vi "GetlastDate.vi"() -> (0 "ResultLine":string, 1 "text":string, 2 "last Date":string, 3 "FRowAsArr":dbl[][](array[numeric]) format="%#_2g")   [LabVIEW 2023]
panel:
  out "result string":string
  out "Array":string[](array[string])
  out "All Officials Result":dbl[][](array[numeric])
  out "First Row":dbl[](array[numeric])
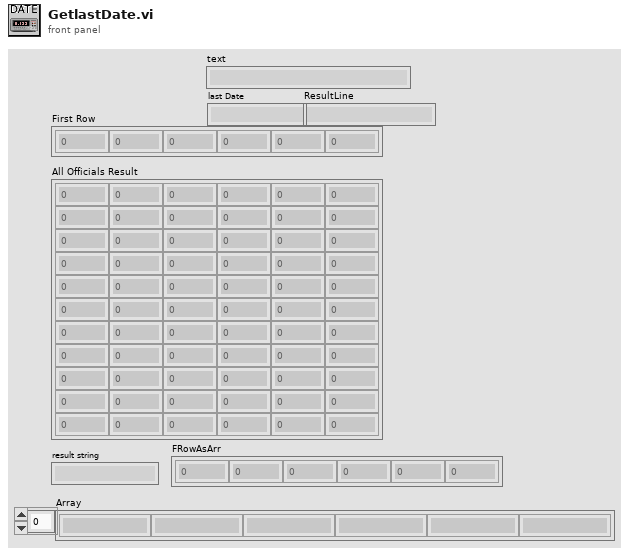
[diagram p1: front panel]
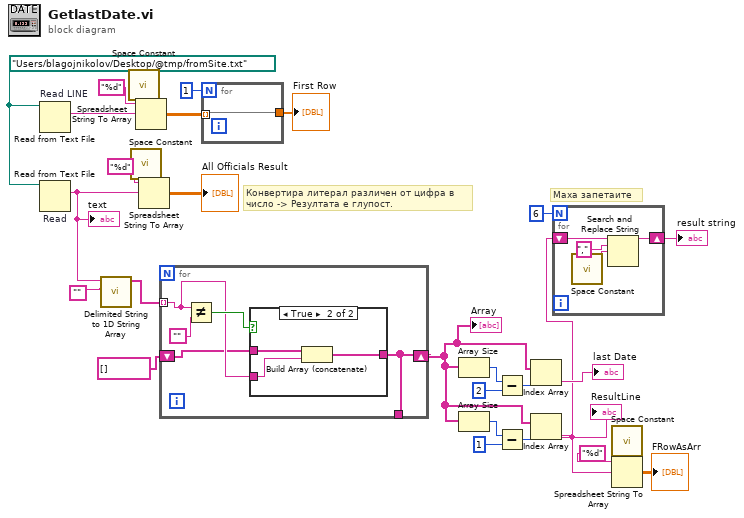
[diagram p0: block diagram]
diagram:
  w20 = path "/Users/blagojnikolov/Desktop/@tmp/fromSite.txt" ("file (use dialog)")
  # "Конвертира литерал различен от цифра в \nчисло -> Резултата е глупост."
  # "Маха запетаите"
  n1 = Read from Text File "Read LINE"(file (use dialog)=w20) -> (text=w28:string)  [unwired: 3 in, 3 out]
  n2 = Read from Text File "Read"(file (use dialog)=w20) -> (text=w18:string)  [unwired: 3 in, 3 out]
  "text" <- w18
  n3 = call <vilib>:"Delimited String to 1D String Array.vi"("delimiter"="", "delimited string"=w18) -> ("string array"=w16:string[])  [unwired: 9 in]
  n4 = call <vilib>:"Space Constant.vi"() -> ("String"=w26:string)
  n5 = call <vilib>:"Space Constant.vi"() -> ("String"=w22:string)
  n6 = Spreadsheet String To Array(delimiter (Tab)=w26, format string="%d", spreadsheet string=w28) -> (array=w25:dbl[][])  [unwired: 1 in]
  n7 = Spreadsheet String To Array(delimiter (Tab)=w22, format string="%d", spreadsheet string=w18) -> (array=→"All Officials Result":dbl[][])  [unwired: 1 in]
  n8 = for {
    tunnel: w16 -> [w31] mode=indexing
    shift-right: [w29] -> w5
    shift-left: string[] [] -> [w30]
    tunnel: [w29] -> _
    n9 = Not Equal?(x=w31, y="") -> (x != y?=w32:bool)
    n10 = case shown="True" w32 {
      tunnel: w31 -> [_ w37]
      tunnel: [w34 w36] -> w29
      tunnel: w30 -> [w34 w35]
      frame False {
      }
      frame True {
        n11 = Build Array (concatenate)(w35, w37) -> (w36:string[])
      }
    }
  }
  "Array" <- w5
  n12 = for {
    N: 1 -> [_]
    tunnel: w25 -> [w38] mode=indexing
    tunnel: [w38] -> w23
  }
  "First Row" <- w23
  n13 = Array Size(array=w5) -> (size(s)=w14:i32)
  n14 = Array Size(array=w5) -> (size(s)=w9:i32)
  n15 = Subtract(x=w14, y=2) -> (x-y=w13:i32)
  n16 = Subtract(x=w9, y=1) -> (x-y=w10:i32)
  n17 = Index Array(array=w5, index=w13) -> (element=→"last Date":string)
  n18 = Index Array(array=w5, index=w10) -> (element=w2:string)
  "ResultLine" <- w2
  n19 = for {
    N: 6 -> [_]
    shift-right: [w40] -> w1
    shift-left: w2 -> [w39]
    n20 = call <vilib>:"Space Constant.vi"() -> ("String"=w41:string)
    n21 = Search and Replace String(input string=w39, search string="," ("replace string (\"\")"), replace string=w41) -> (result string=w40:string)  [unwired: 5 in, 3 out]
  }
  "result string" <- w1
  n22 = call <vilib>:"Space Constant.vi"() -> ("String"=w8:string)
  n23 = Spreadsheet String To Array(delimiter (Tab)=w8, format string="%d", spreadsheet string=w2) -> (array=→"FRowAsArr":dbl[][])  [unwired: 1 in]
